vi "calibrationSpectrometer_issueCommand_CaptureSpectImage.vi"(8 "error in (no error)":errorcluster, 11 "command_CaptureSpectImage_Ctl":T1) -> (0 "error out":errorcluster, 2 "function return":i32, 3 "command_CaptureSpectImage_Ctl out":T1)   [LabVIEW 2016, in "SALLV_calibrationSpectrometer.lvlib"]
doc: "int calibrationSpectrometer_shm_issueCommand_CaptureSpectImageLV(calibrationSpectrometer_command_CaptureSpectImageLV *command_CaptureSpectImage_Ctl );"
uses:
  SALLV_calibrationSpectrometer.lvlib
  DataTypes/command_CaptureSpectImage.ctl
  SALLV_calibrationSpectrometer.so
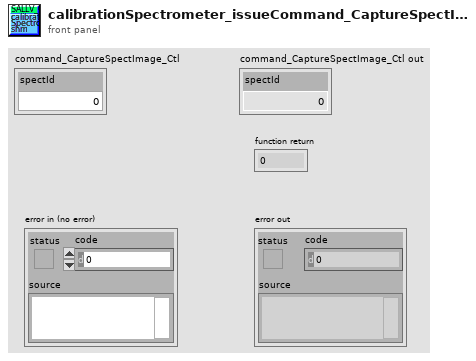
[diagram p1: front panel]
types:
  T1 = typedef "SALLV_calibrationSpectrometer.lvlib/command_CaptureSpectImage.ctl" = cluster{"spectId":u16}
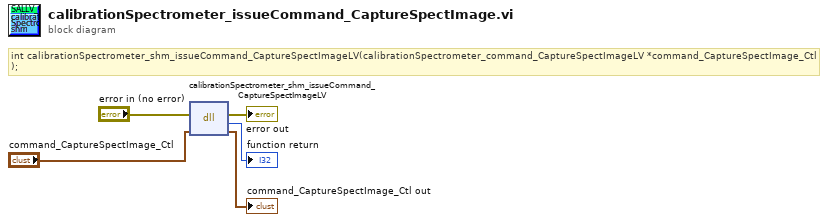
[diagram p0: block diagram]
diagram:
  # "int calibrationSpectrometer_shm_issueCommand_CaptureSpectImageLV(calibrationSpectrometer_command_CaptureSpectImageLV *command_CaptureSpectImage_Ctl );"
  n1 = dll-call lib="home/harini/TCS/sallv_sedspectrometer/SALLV_calibrationSpectrometer.*" fn="calibrationSpectrometer_shm_issueCommand_CaptureSpectImageLV"(error in="error in (no error)", "command_CaptureSpectImage_Ctl"="command_CaptureSpectImage_Ctl") -> (error out=→"error out":errorcluster, →"function return":i32, "command_CaptureSpectImage_Ctl"=→"command_CaptureSpectImage_Ctl out":T1)  [unwired: 2 in, 1 out]
